vi "Izhikevich_coefficients_v001.vi"(8 "Neuron Type":T1(ring)) -> (0 "d":dbl, 1 "c":dbl, 2 "b":dbl, 3 "a":dbl, 4 "u0":dbl, 5 "v0":dbl)   [LabVIEW 2019]
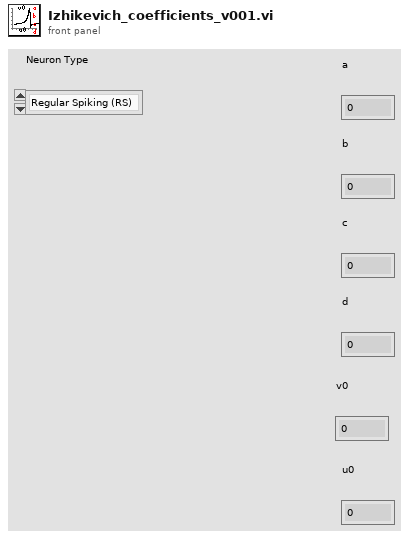
[diagram p1: front panel]
types:
  T1 = enum16{"Regular Spiking (RS)", "Intrinsically Bursting (IB)", "Chattering (CH)", "Fast Spiking (FS)", "Thalamo-Cortical 1 (TC1)", "Thalamo-Cortical 2 (TC2)", "Resonator (RZ)", "Low-Threshold Spiking (LTS)", "Phasic Spiking (PS)"}
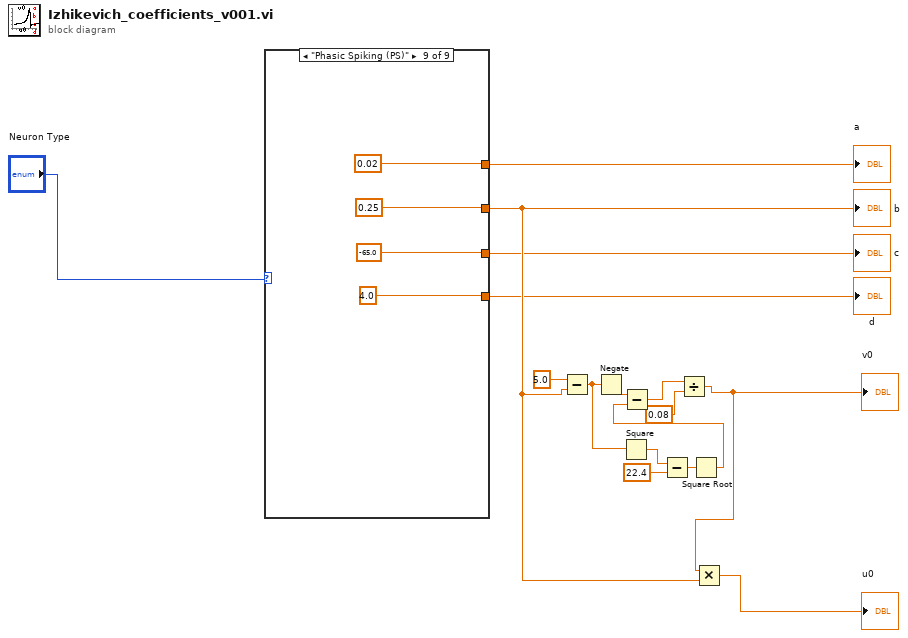
[diagram p0: block diagram]
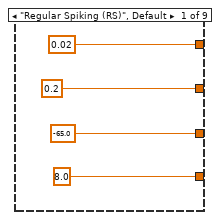
[diagram p2: hidden frame]
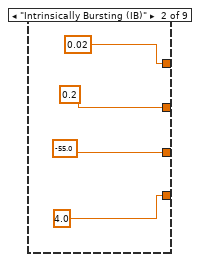
[diagram p3: hidden frame]
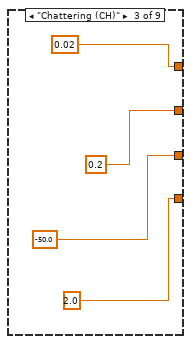
[diagram p4: hidden frame]
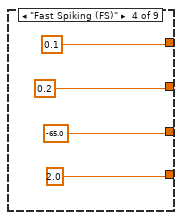
[diagram p5: hidden frame]
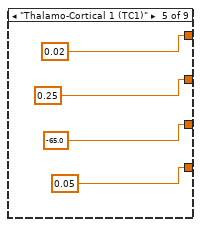
[diagram p6: hidden frame]
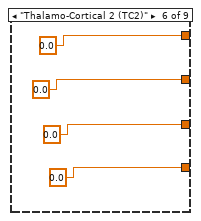
[diagram p7: hidden frame]
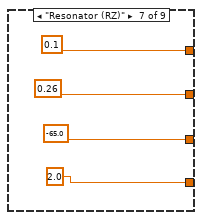
[diagram p8: hidden frame]
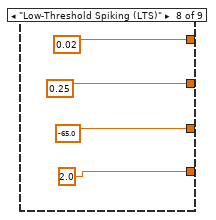
[diagram p9: hidden frame]
diagram:
  n1 = case shown="\"Phasic Spiking (PS)\"" "Neuron Type" {
    tunnel: [0.02 0.02 0.02 0.1 0.02 0.0 0.1 0.02 0.02] -> w2
    tunnel: [0.2 0.2 0.2 0.2 0.25 0.0 0.26 0.25 0.25] -> w15
    tunnel: [-65.0 -55.0 -50.0 -65.0 -65.0 0.0 -65.0 -65.0 -65.0] -> w3
    tunnel: [8.0 4.0 2.0 2.0 0.05 0.0 2.0 2.0 4.0] -> w4
    frame "Regular Spiking (RS)", Default {
    }
    frame "Intrinsically Bursting (IB)" {
    }
    frame "Chattering (CH)" {
    }
    frame "Fast Spiking (FS)" {
    }
    frame "Thalamo-Cortical 1 (TC1)" {
    }
    frame "Thalamo-Cortical 2 (TC2)" {
    }
    frame "Resonator (RZ)" {
    }
    frame "Low-Threshold Spiking (LTS)" {
    }
    frame "Phasic Spiking (PS)" {
    }
  }
  "b" <- w15
  "d" <- w4
  "c" <- w3
  "a" <- w2
  n2 = Subtract(x=5.0, y=w15) -> (x-y=w7:dbl)
  n3 = Negate(x=w7) -> (-x=w6:dbl)
  n4 = Square(x=w7) -> (x^2=w8:dbl)
  n5 = Subtract(x=w8, y=22.4) -> (x-y=w10:dbl)
  n6 = Square Root(x=w10) -> (sqrt(x)=w11:dbl)
  n7 = Subtract(x=w6, y=w11) -> (x-y=w12:dbl)
  n8 = Divide(x=w12, y=0.08) -> (x/y=w14:dbl)
  "v0" <- w14
  n9 = Multiply(x=w14, y=w15) -> (x*y=→"u0":dbl)
